vi "Client Read-Write INI.vi"(8 "error in (no error)":errorcluster, 10 "ServerPort (80)":u16=80, 11 "ServerName (Empty - Read)":string) -> (0 "error out":errorcluster, 1 "Test Timeout (ms)":i32, 2 "ServerPort out":u16=80, 3 "ServerName Out":string)   [LabVIEW 2011]
uses:
  <vilib>/Utility/config.llb/Read Key (I32).vi
  <vilib>/Utility/config.llb/Write Key (String).vi
  <vilib>/Utility/config.llb/Write Key (U32).vi
  <vilib>/Utility/config.llb/Read Key (String).vi
  <vilib>/Utility/config.llb/Read Key (U32).vi
  <vilib>/Utility/config.llb/NI_LVConfig.lvlib
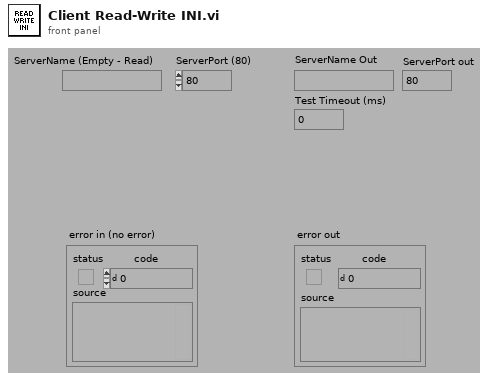
[diagram p1: front panel]
types:
  T1 = enum32{"invalid app kind", "Development System", "Run Time System", "Student Edition", "Embedded LabVIEW", "Evaluation", "Custom"}
  T2 = typedef "NI_LVConfig.lvlib/Config Data RefNum.ctl" = refnum<k1>
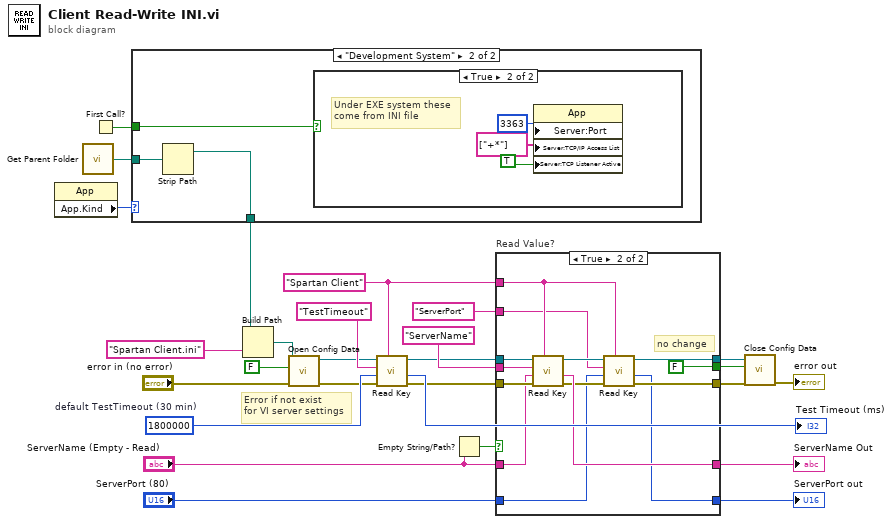
[diagram p0: block diagram]
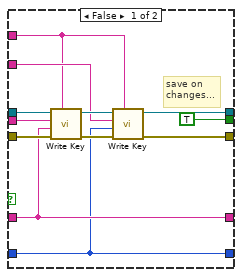
[diagram p2: hidden frame]
diagram:
  w12 = "Spartan Client" ("name or relative path")
  w24 = 1800000  # default TestTimeout (30 min)
  # "Error if not exist\nfor VI server settings"
  n1 = property class="App"() -> ("App.Kind"=w22:T1)  [unwired: 2 in, 2 out]
  n2 = call "Get Parent Folder.vi"() -> ("path"=w8:path)  [unwired: 5 out]
  n3 = First Call?() -> (First Call?: T/F=w4:bool)
  n4 = case shown="\"Development System\"" w22 {
    tunnel: w8 -> [w28 w31]
    tunnel: [w28 w30] -> w5
    tunnel: w4 -> [_ w29]
    frame "invalid app kind", Default {
    }
    frame "Development System" {
      n5 = Strip Path(path=w31) -> (stripped path=w30:path)  [unwired: 1 out]
      n6 = case shown="True" w29 {
        frame False {
        }
        frame True {
          # "Under EXE system these\ncome from INI file"
          n7 = property class="App"("Server:Port"=u32 3363, "Server:TCP/IP Access List"=string[] ["+*"], "Server:TCP Listener Active"=TRUE) -> ()  [unwired: 2 in, 2 out]
        }
      }
    }
  }
  n8 = Build Path(base path=w5, name or relative path="Spartan Client.ini") -> (appended path=w6:path)
  n9 = call <vilib>:"Open Config Data.vi"("error in (no error)"="error in (no error)", "create file if necessary (T)"=FALSE, "configuration file path"=w6) -> ("error out"=w15:errorcluster, "refnum"=w11:T2)  [unwired: 6 in, 1 out]
  n10 = call-poly <vilib>:"Read Key.vi"("section"=w12, "error in (no error)"=w15, "default value"=w24, "key"="TestTimeout" ("name or relative path"), "refnum"=w11) -> ("error out"=w14:errorcluster, "value"=→"Test Timeout (ms)":i32, "refnum out"=w13:T2)  [unwired: 4 out]
  n11 = Empty String/Path?(string/path="ServerName (Empty - Read)") -> (empty?=w18:bool)
  n12 = case "Read Value?" shown="True" w18 {
    tunnel: w14 -> [w45 w60]
    tunnel: w12 -> [w36 w50]
    tunnel: w13 -> [w46 w59]
    tunnel: "ServerName" ("name or relative path") -> [w44 w58]
    tunnel: [w39 w52] -> w20
    tunnel: [w38 w51] -> w19
    tunnel: "ServerName (Empty - Read)" -> [w43 w57]
    tunnel: [w43 w56] -> w25
    tunnel: [TRUE FALSE] -> w16
    tunnel: "ServerPort (80)" -> [w35 w48]
    tunnel: "ServerPort" ("name or relative path") -> [w37 w49]
    tunnel: [w35 w47] -> w1
    frame False {
      # "save on\nchanges..."
      n13 = call-poly <vilib>:"Write Key.vi"("section"=w36, "error in (no error)"=w45, "value"=w43, "key"=w44, "refnum"=w46) -> ("error out"=w40:errorcluster, "refnum out"=w41:T2)  [unwired: 1 in, 4 out]
      n14 = call-poly <vilib>:"Write Key.vi"("section"=w36, "error in (no error)"=w40, "value"=w35, "key"=w37, "refnum"=w41) -> ("error out"=w38:errorcluster, "refnum out"=w39:T2)  [unwired: 5 out]
    }
    frame True {
      # "no change"
      n15 = call-poly <vilib>:"Read Key.vi"("section"=w50, "error in (no error)"=w60, "default value"=w57, "key"=w58, "refnum"=w59) -> ("error out"=w53:errorcluster, "value"=w56:string, "refnum out"=w54:T2)  [unwired: 1 in, 3 out]
      n16 = call-poly <vilib>:"Read Key.vi"("section"=w50, "error in (no error)"=w53, "default value"=w48, "key"=w49, "refnum"=w54) -> ("error out"=w51:errorcluster, "value"=w47:u32, "refnum out"=w52:T2)  [unwired: 4 out]
    }
  }
  "ServerName Out" <- w25
  "ServerPort out" <- w1
  n17 = call <vilib>:"Close Config Data.vi"("error in (no error)"=w19, "write file if changed (T)"=w16, "refnum"=w20) -> ("error out"=→"error out":errorcluster)  [unwired: 8 out]
